vi "C(T) Elvis FG control.vi"(0 "Device Name":tag="Dev1", 1 "Stop":bool, 2 "Frequency (Hz)":dbl=43.0 min=0.2 max=5000000.0 step=0.1 format="%#.2p", 3 "DC Offset (V)":dbl min=-5.0 max=5.0 format="%.2p", 4 "Amplitude (Vpp)":dbl=0.05 min=0.0 max=10.0 step=0.01 format="%#.2p", 5 "error in":errorcluster, 7 "Type":u16(ring) items=["Sine", "Triangle", "Square"], 8 "Manual":bool, 10 "Signal Route":u16(ring) items=["Prototyping board", "FGEN BNC", "AO 0"], 11 "Duty Cycle (%)":dbl=50.0 min=0.0 max=100.0 step=1.0) -> (16 "Manual?":bool, 19 "error out":errorcluster)   [LabVIEW 2016]
doc: "This VI sets to ELVIS FG to generate the 43 Hz square wave on SYNC OUT to drive the C(T) experiment.\n\nPaul K Dixon\nPhysics 350\nCSUSB Physics"
uses:
  <vilib>/express/NI ELVISmx/misc.llb/ctl_ProductType.ctl
  <resource>/objmgr/daqmx.rc
  nilvaiu.dll
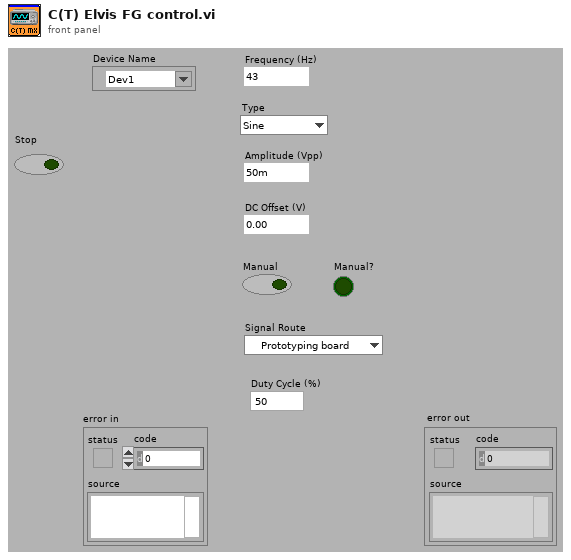
[diagram p1: front panel]
types:
  T1 = typedef "ctl_ProductType.ctl" = enum16{"NI myDAQ", "NI ELVIS II", "NI ELVIS II+"}
  T2 = cluster{"Duty Cycle (%)":dbl, "Type":u16, "Frequency (Hz)":dbl, "Amplitude":dbl, "DC Offset (V)":dbl}
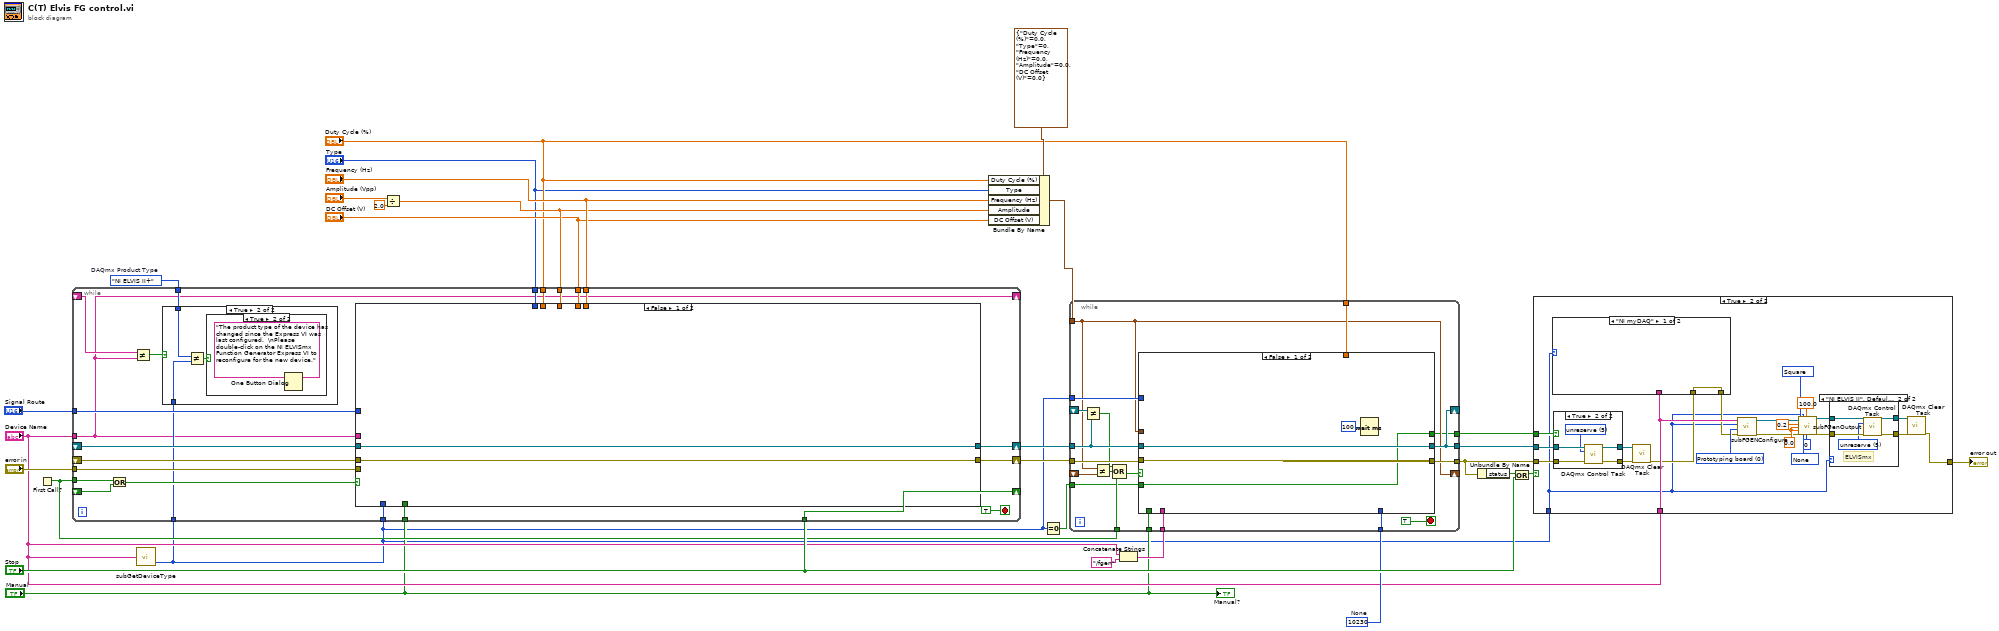
[diagram p0: block diagram]
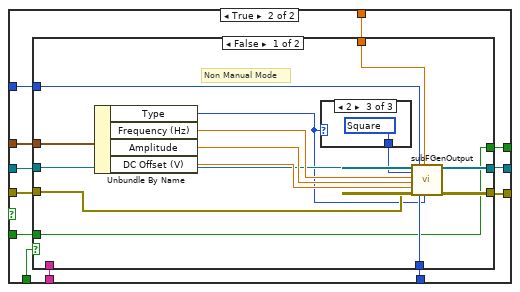
[diagram p2: hidden frame]
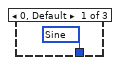
[diagram p3: hidden frame]
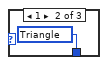
[diagram p4: hidden frame]
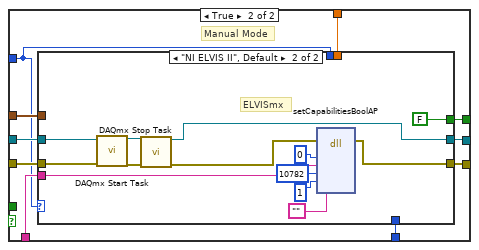
[diagram p5: hidden frame]
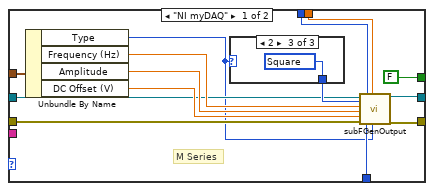
[diagram p6: hidden frame]
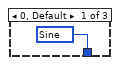
[diagram p7: hidden frame]
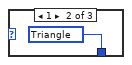
[diagram p8: hidden frame]
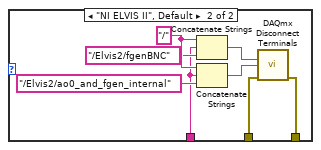
[diagram p10: hidden frame]
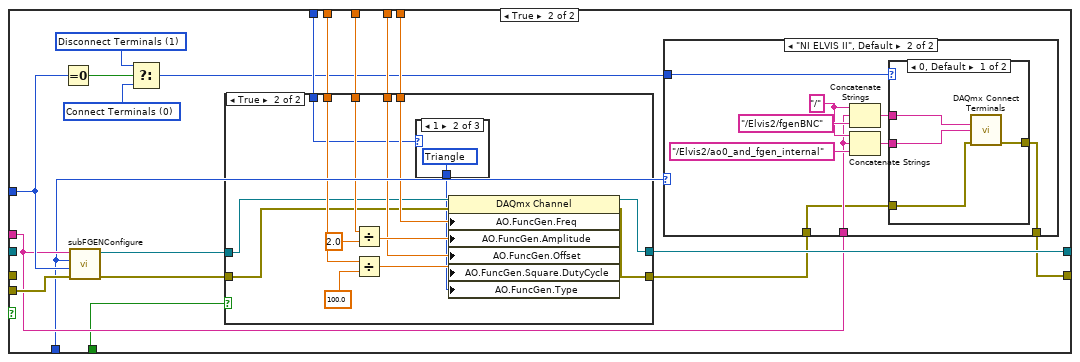
[diagram p15: hidden frame]
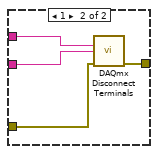
[diagram p17: hidden frame]
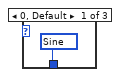
[diagram p19: hidden frame]
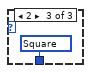
[diagram p20: hidden frame]
diagram:
  w13 = 10230  # None
  w2 = ctl_ProductType."NI ELVIS II+"  # DAQmx Product Type
  n1 = First Call?() -> (First Call?: T/F=w23:bool)
  n2 = call <vilib>:"subGetDeviceType.vi"("DAQmx Device Name"="Device Name") -> ("Product Type"=w1:T1)  [unwired: 3 in, 1 out]
  n3 = Divide(x="Amplitude (Vpp)", y=2.0) -> (x/y=w6:dbl)
  n4 = while {
    shift-right: [w52] -> w20
    shift-left: _ -> [w50]
    shift-right: [w47] -> _
    shift-left: _ -> [w43]
    tunnel: "Stop" -> [w47]
    tunnel: w23 -> [w41]
    tunnel: "error in" -> [w49]
    shift-right: [w51] -> w21
    shift-left: _ -> [w45]
    tunnel: "Device Name" -> [w31]
    tunnel: w1 -> [w44]
    tunnel: "Signal Route" -> [w42]
    tunnel: "Manual" -> [w40]
    tunnel: "Frequency (Hz)" -> [w39]
    tunnel: w6 -> [w38]
    tunnel: "DC Offset (V)" -> [w37]
    tunnel: "Duty Cycle (%)" -> [w36]
    tunnel: "Type" -> [w35]
    tunnel: w2 -> [w34]
    tunnel: w1 -> [w33]
    shift-right: [w31] -> _
    shift-left: _ -> [w32]
    stop <- TRUE stop-if-true
    n5 = Or(x=w41, y=w43) -> (x .or. y?=w46:bool)
    n6 = Not Equal?(x=w32, y=w31) -> (x != y?=w30:bool)
    n7 = case shown="True" w30 {
      tunnel: w34 -> [_ w55]
      tunnel: w33 -> [_ w53]
      frame False {
      }
      frame True {
        n8 = Not Equal?(x=w55, y=w53) -> (x != y?=w54:bool)
        n9 = case shown="True" w54 {
          frame False {
          }
          frame True {
            n10 = One Button Dialog(message="The product type of the device has changed since the Express VI was last configured.  \nPlease double-click on the NI ELVISmx Function Generator Express VI to reconfigure for the new device.") -> ()  [unwired: 1 in, 1 out]
          }
        }
      }
    }
    n11 = case shown="False" w46 {
      tunnel: [w58 w70] -> w52
      tunnel: [w57 w61] -> w51
      tunnel: w50 -> [w58 _]
      tunnel: w49 -> [_ w77]
      tunnel: w45 -> [w57 _]
      tunnel: w31 -> [_ w64]
      tunnel: w44 -> [_ w60]
      tunnel: w42 -> [_ w73]
      tunnel: w40 -> [_ w59]
      tunnel: w39 -> [_ w69]
      tunnel: w38 -> [_ w68]
      tunnel: w37 -> [_ w67]
      tunnel: w36 -> [_ w66]
      tunnel: w35 -> [_ w65]
      frame False {
      }
      frame True {
        w76 = u16 0 items=["Connect Terminals", "Disconnect Terminals"] ("Action")
        w75 = u16 1 items=["Connect Terminals", "Disconnect Terminals"] ("Action")
        n12 = Equal To 0?(x=w73) -> (x = 0?=w74:bool)
        n13 = call <vilib>:"subFGENConfigure.vi"("error in"=w77, "Signal Route"=w73, "Device Type"=w60, "DAQmx Device Name"=w64) -> ("error out"=w72:errorcluster, "task out"=w71:refnum<k21>)  [unwired: 6 in]
        n14 = Select(t=w75, s=w74, f=w76) -> (s? t:f=w62:u16)
        n15 = case shown="True" w59 {
          tunnel: w72 -> [w97 w102]
          tunnel: [w97 w100] -> w63
          tunnel: w71 -> [w96 w103]
          tunnel: [w96 w101] -> w70
          tunnel: w69 -> [_ w107]
          tunnel: w68 -> [_ w106]
          tunnel: w67 -> [_ w105]
          tunnel: w66 -> [_ w104]
          tunnel: w65 -> [_ w99]
          frame False {
          }
          frame True {
            n16 = Divide(x=w106, y=2.0) -> (x/y=w108:dbl)
            n17 = Divide(x=w104, y=100.0) -> (x/y=w109:dbl)
            n18 = case shown="1" w99 {
              tunnel: [w112 w113 w114] -> w98
              frame 0, Default {
                w112 = 14751 items=["Sine"=14751, "Triangle"=14752, "Square"=14753, "Sawtooth"=14754] ("AO.FuncGen.Type")
              }
              frame 1 {
                w113 = 14752 items=["Sine"=14751, "Triangle"=14752, "Square"=14753, "Sawtooth"=14754] ("AO.FuncGen.Type")
              }
              frame 2 {
                w114 = 14753 items=["Sine"=14751, "Triangle"=14752, "Square"=14753, "Sawtooth"=14754] ("AO.FuncGen.Type")
              }
            }
            n19 = property class="DAQmx Channel"(reference=w103, error in=w102, "AO.FuncGen.Freq"=w107, "AO.FuncGen.Amplitude"=w108, "AO.FuncGen.Offset"=w105, "AO.FuncGen.Square.DutyCycle"=w109, "AO.FuncGen.Type"=w98) -> (reference out=w101:refnum<k21>, error out=w100:errorcluster)
          }
        }
        n20 = case shown="\"NI ELVIS II\", Default" w60 {
          tunnel: w64 -> [_ w82]
          tunnel: w63 -> [w78 w81]
          tunnel: w62 -> [_ w80]
          tunnel: [w78 w79] -> w61
          frame "NI myDAQ" {
          }
          frame "NI ELVIS II", Default {
            w83 = "/"
            n21 = Concatenate Strings(w83, w82, "/Elvis2/fgenBNC" ("string")) -> (w86:string)
            n22 = Concatenate Strings(w83, w82, "/Elvis2/ao0_and_fgen_internal" ("string")) -> (w87:string)
            n23 = case shown="0, Default" w80 {
              tunnel: w86 -> [w91 w95]
              tunnel: w87 -> [w90 w94]
              tunnel: [w89 w93] -> w79
              tunnel: w81 -> [w88 w92]
              frame 0, Default {
                n24 = call <vilib>:"DAQmx Connect Terminals.vi"("source terminal"=w91, "destination terminal"=w90, "error in"=w88) -> ("error out"=w89:errorcluster)  [unwired: 12 in]
              }
              frame 1 {
                n25 = call <vilib>:"DAQmx Disconnect Terminals.vi"("source terminal"=w95, "destination terminal"=w94, "error in"=w92) -> ("error out"=w93:errorcluster)  [unwired: 12 in]
              }
            }
          }
        }
      }
    }
  }
  n26 = Bundle By Name(cluster=T2 {"Duty Cycle (%)"=0.0, "Type"=0, "Frequency (Hz)"=0.0, "Amplitude"=0.0, "DC Offset (V)"=0.0} ("output cluster"), "Duty Cycle (%)"="Duty Cycle (%)", "Type"="Type", "Frequency (Hz)"="Frequency (Hz)", "Amplitude"=w6, "DC Offset (V)"="DC Offset (V)") -> (w11:T2)
  n27 = Equal To 0?(x=w1) -> (x = 0?=w17:bool)
  n28 = Concatenate Strings("Device Name", "/fgen" ("string")) -> (w18:string)
  n29 = while {
    tunnel: [w122] -> w29
    tunnel: [w133] -> w22
    tunnel: w20 -> [w121]
    tunnel: w21 -> [w132]
    shift-right: [w117] -> _
    shift-left: _ -> [w116]
    tunnel: w11 -> [w117]
    tunnel: w23 -> [w131]
    tunnel: w13 -> [w127]
    tunnel: w18 -> [w126]
    tunnel: w17 -> [w125]
    tunnel: w1 -> [w124]
    tunnel: "Manual" -> [w123]
    shift-right: [w122] -> _
    shift-left: _ -> [w120]
    tunnel: "Duty Cycle (%)" -> [w118]
    tunnel: [w115] -> w10
    stop <- TRUE stop-if-true
    n30 = Not Equal?(x=w120, y=w121) -> (x != y?=w119:bool)
    n31 = Not Equal?(x=w117, y=w116) -> (x != y?=w128:bool)
    n32 = Compound Arithmetic op=OR(w119, w128, w131) -> (w130:bool)
    n33 = case shown="False" w130 {
      tunnel: [w137 w144] -> w122
      tunnel: [w136 w143] -> w133
      tunnel: w121 -> [w137 w148]
      tunnel: w132 -> [w136 w147]
      tunnel: w117 -> [_ w149]
      tunnel: w127 -> [_ w145]
      tunnel: w126 -> [_ w146]
      tunnel: w125 -> [w134 w142]
      tunnel: w124 -> [_ w141]
      tunnel: w123 -> [_ w140]
      tunnel: w118 -> [_ w139]
      tunnel: [w134 w138] -> w115
      frame False {
        n34 = Wait (ms)(milliseconds to wait=u32 100) -> ()  [unwired: 1 out]
      }
      frame True {
        n35 = case "Manual" shown="False" w140 {
          tunnel: w149 -> [w160 w171]
          tunnel: w148 -> [w159 w173]
          tunnel: w147 -> [w158 w176]
          tunnel: w146 -> [_ w174]
          tunnel: w145 -> [w157 w170]
          tunnel: [w156 w172] -> w144
          tunnel: [w155 w175] -> w143
          tunnel: w142 -> [w150 _]
          tunnel: w141 -> [w153 w167]
          tunnel: w139 -> [w151 w169]
          tunnel: [w150 w168] -> w138
          frame False {
            # "Non Manual Mode"
            n36 = Unbundle By Name(w160) -> ("Type"=w152:u16, "Frequency (Hz)"=w161:dbl, "Amplitude"=w162:dbl, "DC Offset (V)"=w163:dbl)
            n37 = case shown="2" w152 {
              tunnel: [w164 w165 w166] -> w154
              frame 0, Default {
                w164 = 14751 items=["Sine"=14751, "Triangle"=14752, "Square"=14753, "Sawtooth"=14754] ("AO.FuncGen.Type")
              }
              frame 1 {
                w165 = 14752 items=["Sine"=14751, "Triangle"=14752, "Square"=14753, "Sawtooth"=14754] ("AO.FuncGen.Type")
              }
              frame 2 {
                w166 = 14753 items=["Sine"=14751, "Triangle"=14752, "Square"=14753, "Sawtooth"=14754] ("AO.FuncGen.Type")
              }
            }
            n38 = call <vilib>:"subFGenOutput.vi"("task in"=w159, "AO.FuncGen.Type"=w154, "Frequency"=w161, "Amplitude"=w162, "Offset"=w163, "error in (no error)"=w158, "Device Type"=w153, "AO.FuncGen.ModulationType"=w157, "square wave duty cycle (%)"=w151, "Signal Type"=w152) -> ("task out"=w156:refnum<k21>, "error out"=w155:errorcluster)  [unwired: 7 in, 1 out]
          }
          frame True {
            # "Manual Mode"
            n39 = case shown="\"NI ELVIS II\", Default" w167 {
              tunnel: w176 -> [w182 w206]
              tunnel: [w184 w194] -> w175
              tunnel: w174 -> [_ w196]
              tunnel: w173 -> [w183 w203]
              tunnel: [w185 w204] -> w172
              tunnel: w171 -> [w186 _]
              tunnel: w167 -> [w181 _]
              tunnel: w170 -> [w180 _]
              tunnel: w169 -> [w178 _]
              tunnel: [FALSE FALSE] -> w168
              frame "NI myDAQ" {
                # "M Series"
                n40 = Unbundle By Name(w186) -> ("Type"=w179:u16, "Frequency (Hz)"=w188:dbl, "Amplitude"=w189:dbl, "DC Offset (V)"=w190:dbl)
                n41 = case shown="2" w179 {
                  tunnel: [w191 w192 w193] -> w187
                  frame 0, Default {
                    w191 = 14751 items=["Sine"=14751, "Triangle"=14752, "Square"=14753, "Sawtooth"=14754] ("AO.FuncGen.Type")
                  }
                  frame 1 {
                    w192 = 14752 items=["Sine"=14751, "Triangle"=14752, "Square"=14753, "Sawtooth"=14754] ("AO.FuncGen.Type")
                  }
                  frame 2 {
                    w193 = 14753 items=["Sine"=14751, "Triangle"=14752, "Square"=14753, "Sawtooth"=14754] ("AO.FuncGen.Type")
                  }
                }
                n42 = call <vilib>:"subFGenOutput.vi"("task in"=w183, "AO.FuncGen.Type"=w187, "Frequency"=w188, "Amplitude"=w189, "Offset"=w190, "error in (no error)"=w182, "Device Type"=w181, "AO.FuncGen.ModulationType"=w180, "square wave duty cycle (%)"=w178, "Signal Type"=w179) -> ("task out"=w185:refnum<k21>, "error out"=w184:errorcluster)  [unwired: 7 in, 1 out]
              }
              frame "NI ELVIS II", Default {
                # "ELVISmx"
                n43 = call <vilib>:"DAQmx Start Task.vi"("task/channels in"=w203, "error in"=w206) -> ("task out"=w202:refnum<k21>, "error out"=w205:errorcluster)  [unwired: 12 in]
                n44 = call <vilib>:"DAQmx Stop Task.vi"("task/channels in"=w202, "error in"=w205) -> ("task out"=w204:refnum<k21>, "error out"=w195:errorcluster)  [unwired: 12 in]
                n45 = dll-call lib="nilvaiu.dll" fn="setCapabilitiesBoolAP"(error in=w195, "taskID"=u32 0, "activeProperty"=w196, "attributeID"=10782, "paramValue"=1, "extendedErrorInfoHdlPtr"="" ("Empty String Constant")) -> (error out=w194:errorcluster)  [unwired: 8 in, 1 out]
              }
            }
          }
        }
      }
    }
  }
  n46 = Unbundle By Name(w22) -> ("status"=w27:bool)
  n47 = Or(x=w27, y="Stop") -> (x .or. y?=w26:bool)
  n48 = case shown="True" w26 {
    tunnel: w29 -> [_ w227]
    tunnel: w22 -> [w207 w229]
    tunnel: [w207 w209] -> w28
    tunnel: w10 -> [_ w230]
    tunnel: "Device Name" -> [_ w225]
    tunnel: w1 -> [_ w208]
    frame False {
    }
    frame True {
      w212 = 14753 items=["Sine"=14751, "Triangle"=14752, "Square"=14753, "Sawtooth"=14754] ("AO.FuncGen.Type")
      w216 = 10230 items=["AM"=14756, "FM"=14757, "None"=10230] ("AO.FuncGen.ModulationType")
      w215 = 0.0 ("Amplitude")
      w224 = u16 0 items=["Prototyping board", "FGEN BNC"] ("Signal Route")
      n49 = case shown="True" w230 {
        tunnel: w229 -> [w247 w253]
        tunnel: [w247 w252] -> w228
        tunnel: w227 -> [w248 w251]
        tunnel: [w248 w250] -> w226
        frame False {
        }
        frame True {
          w249 = 5 items=["verify"=2, "reserve"=4, "commit"=3, "unreserve"=5, "abort"=6] ("action")
          n50 = call <vilib>:"DAQmx Control Task.vi"("task/channels in"=w251, "action"=w249, "error in"=w253) -> ("task out"=w250:refnum<k21>, "error out"=w252:errorcluster)  [unwired: 11 in]
        }
      }
      n51 = call <vilib>:"DAQmx Clear Task.vi"("task in"=w226, "error in"=w228) -> ("error out"=w223:errorcluster)  [unwired: 13 in]
      n52 = case shown="\"NI myDAQ\"" w208 {
        tunnel: w225 -> [_ w234]
        tunnel: w223 -> [w231 w233]
        tunnel: [w231 w232] -> w222
        frame "NI myDAQ" {
        }
        frame "NI ELVIS II", Default {
          w237 = "/"
          n53 = Concatenate Strings(w237, w234, "/Elvis2/fgenBNC" ("string")) -> (w238:string)
          n54 = Concatenate Strings(w237, w234, "/Elvis2/ao0_and_fgen_internal" ("string")) -> (w239:string)
          n55 = call <vilib>:"DAQmx Disconnect Terminals.vi"("source terminal"=w238, "destination terminal"=w239, "error in"=w233) -> ("error out"=w232:errorcluster)  [unwired: 12 in]
        }
      }
      n56 = call <vilib>:"subFGENConfigure.vi"("error in"=w222, "Signal Route"=w224, "Device Type"=w208, "DAQmx Device Name"=w225) -> ("error out"=w210:errorcluster, "task out"=w211:refnum<k21>)  [unwired: 6 in]
      n57 = call <vilib>:"subFGenOutput.vi"("task in"=w211, "AO.FuncGen.Type"=w212, "Frequency"=0.2, "Amplitude"=w215, "Offset"=w215, "error in (no error)"=w210, "Device Type"=w208, "AO.FuncGen.ModulationType"=w216, "square wave duty cycle (%)"=100.0, "Signal Type"=0) -> ("task out"=w218:refnum<k21>, "error out"=w219:errorcluster)  [unwired: 7 in, 1 out]
      n58 = case shown="\"NI ELVIS II\", Default" w208 {
        tunnel: [w241 w246] -> w221
        tunnel: [w240 w245] -> w220
        tunnel: w219 -> [w240 w244]
        tunnel: w218 -> [w241 w243]
        frame "NI myDAQ" {
          # "M Series"
        }
        frame "NI ELVIS II", Default {
          w242 = 5 items=["verify"=2, "reserve"=4, "commit"=3, "unreserve"=5, "abort"=6] ("action")
          # "ELVISmx"
          n59 = call <vilib>:"DAQmx Control Task.vi"("task/channels in"=w243, "action"=w242, "error in"=w244) -> ("task out"=w246:refnum<k21>, "error out"=w245:errorcluster)  [unwired: 11 in]
        }
      }
      n60 = call <vilib>:"DAQmx Clear Task.vi"("task in"=w221, "error in"=w220) -> ("error out"=w209:errorcluster)  [unwired: 13 in]
    }
  }
  "error out" <- w28
  "Manual?" <- "Manual"
